vi "Test Not In Process Loop When Initialized.vi"(8 "error in (no error)":errorcluster, 11 "Test Case In":refnum<class "Process Lifecycle Test.lvclass">) -> (0 "error out":errorcluster, 3 "Test Case Out":refnum<class "Process Lifecycle Test.lvclass">)   [LabVIEW 2020, in "Process Lifecycle Test.lvclass"]
uses:
  Process Lifecycle Test.lvclass
  Process Lifecycle Test.lvclass/Process Lifecycle Test.ctl
  source/Framework/Process/Process.lvclass
  936c6dff-2bd7-4b00-9edb-c16dad16380d.vi
  source/Framework/Process/Public/Lifecycle/API Mode.ctl
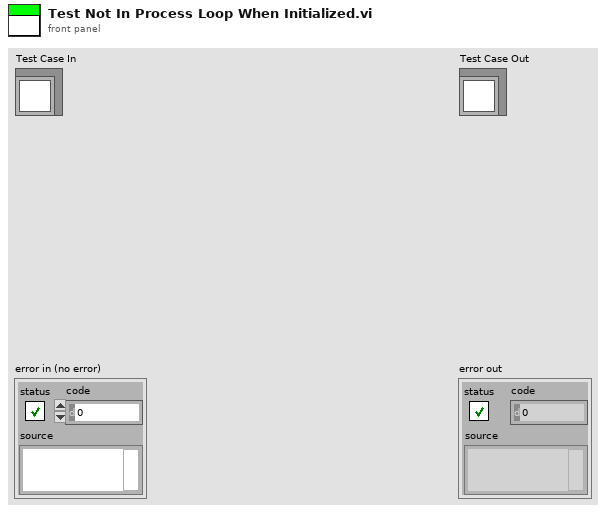
[diagram p1: front panel]
types:
  T1 = typedef "Process.lvclass/API Mode.ctl" = enum16{"Send Message", "Handle Message"}
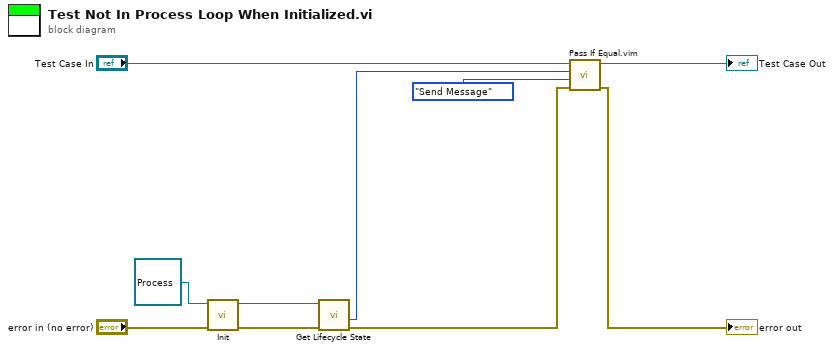
[diagram p0: block diagram]
diagram:
  n1 = call-dynamic "Init.vi"("error in (no error)"="error in (no error)", "Process In"=refnum<class "Process.lvclass"> refnum) -> ("error out"=w4:errorcluster, "Process Out"=w2:refnum<class "Process.lvclass">)  [unwired: 8 in]
  n2 = call "Get Lifecycle State.vi"("error in (no error)"=w4, "Process In"=w2) -> ("error out"=w6:errorcluster, "API Mode"=w5:T1)  [unwired: 6 in, 2 out]
  n3 = call "Pass If Equal.vim"("error in (no error)"=w6, "Actual"=API_Mode."Send Message" ("API Mode"), "Expected"=w5, "LUnit Test Case In"="Test Case In") -> ("error out"=→"error out":errorcluster, "LUnit Test Case Out"=→"Test Case Out":refnum<class "Process Lifecycle Test.lvclass">)  [unwired: 6 in]
